vi "显示图片.vi"(0 "路径":path=path "D:/毕业设计/程序/客户端程序/和风天气图标/未知.png" caption="PNG文件路径", 3 "缩放因子":dbl=1.0) -> (7 "二维图片":T1 caption="显示图片")   [LabVIEW 2016]
uses:
  <vilib>/regexp/Match Regular Expression.xnode
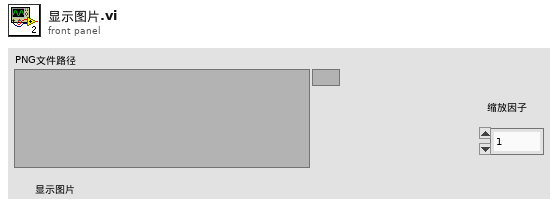
[diagram p1: front panel]
types:
  T1 = typedef "透明背景.ctl" = picture
  T2 = typedef "imagedata.ctl" = cluster{"image type":i32, "image depth":i32, "image":u8[], "mask":u8[], "colors":u32[], "Rectangle":cluster{"left":i16, "top":i16, "right":i16, "bottom":i16}}
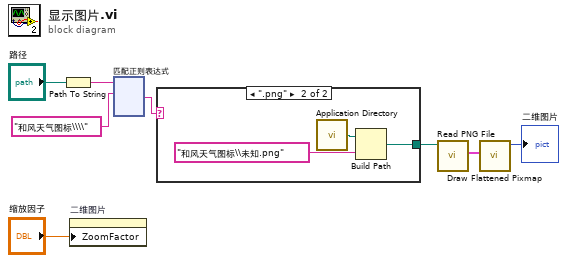
[diagram p0: block diagram]
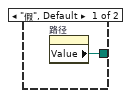
[diagram p2: hidden frame]
diagram:
  n1 = Path To String(path="路径") -> (string=w4:string)
  n2 = property on="二维图片" class="Pict (严格)"("ZoomFactor"="缩放因子") -> ()  [unwired: 2 in, 2 out]
  n3 = xnode "匹配正则表达式"("输入字符串"=w4, "正则表达式"="和风天气图标\\\\") -> ("匹配之后"=w2:string)  [unwired: 4 in, 4 out]
  n4 = case shown="\".png\"" w2 {
    tunnel: [w9 w12] -> w1
    frame "假", Default {
      n5 = property on="路径" class="Path"() -> ("Value"=w9:path)  [unwired: 2 in, 2 out]
    }
    frame ".png" {
      n6 = call <vilib>:"Application Directory.vi"() -> ("Application Directory"=w11:path)
      n7 = Build Path(base path=w11, name or relative path="和风天气图标\\未知.png" ("名称或相对路径")) -> (appended path=w12:path)
    }
  }
  n8 = call <vilib>:"Read PNG File.vi"("path to PNG file"=w1) -> ("image data"=w8:T2)  [unwired: 8 in, 2 out]
  n9 = call <vilib>:"Draw Flattened Pixmap.vi"("image data"=w8) -> ("new picture"=→"二维图片":picture)  [unwired: 8 in]
